vi "Day 10-2.vi"() -> ()   [LabVIEW 2019, in "Day 10.lvlib"]
uses:
  Day 10.lvlib
panel:
  out "Result":u64
  in  "String":string="[[{(<({[(([[([()<>][()<>])]][<{[[]<>]}<<[]{}>>>])[({<[{}[]]<{}<>>><{()[]}[{}[]]>}<<(<>[])[[]{}]>{(<\n{{{[[<{<{({({(<>{})}<(()[])([]<>)>)})(<[([{}()]([]{}))[([][])([]<>)]]((<{}<>>[[]{}])({<>()}{()}))>\n[(<<[(<[[[<{(([]{})){<{}{}>{()<>}})><(<[()()][<>]>([[]]))[(([]<>)(<><>))((<>)({}[]))]>]{<<{{()[]}<[]<>>}\n{{({{{([<((<[[<>[]](<>[])]><<(()<>)<<><>>>{(()<>)(<>{})}>))>]({(([{{()()}>{{{}{}}{<><>}}]{({()<>\n<<{(<<{<<{([{{(){}}{()()}}{<[]{}>(<>{}))][({<>{}}[[]<>])<{{}{}}{{}()}>])[<<{{}{}}[()[]]>{{\n[[<{[<((<[[{{{{}{}}{{}[]}}}[[<{}<>>]]]({<([][]){{}<>}>((()<>)<<>[]>)})]><[({{<{}()>{()()}}})]{(<({[]{}}[{\n<<[{([[[[[<{[([]())({}[])]{[{}[]]}}<(<[]{}>({}{})){{[]<>}[()]}>>{(<{[]}[<>[]]>)}][(([[{}[]]<[]\n[(<[<{{((<{<[<{}[]>[<>{}]][<{}<>>]><<({}[])[[]<>]>}}>)<(([{<{}<>>(()[])}[[{}()]([])]]<<{<>()}({}{})>\n<{{[[<(<<<([({{}())([]{})){<()<>>{<>{}}}]<{[[]{}][[]<>]}{<{}()>{[]()}}>)<<{(<>())[<><>]}[{{}[]}(<>(\n{{{{<{{<{<<[[[{}()]<[][])]<{(){}}{[]{}}>][{<[]()>{<>{}}}]>><{(<<<>[]>{(){}}>{{[]()}[<><>]}){(<{}()>){[[][]](\n{(<{{([[(<{[((()<>){()()})<[<>{}]{()}>]<{[()[]]}>}([{<()>{{}[]}}[([][]){()[]}]]{{<<>[]>}{([]{}){<><>}}})\n[(((({[{<<{[{([]())(<>[])}[<{}()>{()()}]]}>>[<[[{{{}()}{()<>}}(<()<>>[{}[]])]{[({}<>)<<>>]}]<({<<><>\n<([[[((<[<<((<[][]>))<<{[][]}>>>{<([()()>)>}><([[[()[]]({}())]({<>{}}{()[]})]{{{<><>}[[]()]}[[[]\n(((<({([[({{({[][]})(({}())[()<>])}(<[[][]]>(<{}>[<>{}]))})](<{((<<><>>[()()]){<[]<>>[[]<>]})}([<\n[[{[[{[[{[{{[<{}()><()[]>]}}]<<{{<<><>>{{}{}}}[(<>{})(()())]}[{([]<>)[{}()]}<[[]][()()]>]><<{{[]{}}\n((<<((<(<[{[({()<>}{()()}){<{}{}>}]}[{<[<>()][[]()]>}]]{[{[<()>{[]{}}]}<{[{}{}}}[([]{})(<><>)]>](({(<>{})\n[[<[<({[[<<{[[()()]{(){}}]<[{}<>](()())>>(<[()[]][[]()]>)>[{(([][])([]{}))}[<<<><>><()<>>>(<<>[]>)]\n[({(<{(<{[{[{([]){{}{}}}(<[][]>(<>[]))](<{<>[]}<[]()>>{<()><{}>})}{[([<>{}]{[]()})[(<>{})<[]()>]][{[()<>\n[[<<{[(<({(((([]{})[[][]])<<{}{}>{[]()}>))})<[(<<(<>[])<[]()>><((){})[()<>]>>{<({}[])>{<<>{}>{(){}}}}\n<<([[({(<{<[[({}()){()[]}]]>((<<()[]>(<>{})>(([]())))(((()<>)({}[]))))}>{<{((([])<()[]>)<({}())<()<\n<<({[<{<({{{{[()()]<<>[]>}[{{}<>}[()()]]}{(([]()))})})[[[{[<<>[]>[<>()]]<{[]{}}[<>{}]>}]([{{[][]}{\n{((((([[([<{([<>{}]<{}[]>){({}())[{}[]]}}{(<()()>({}[]))<{<><>}(<>[])>}>([<{()<>}[()[]]><[()<>]>]{[{\n{[((((({<[{<{[(){}][[]()]}[({}[])]>{[[<>{}]{{}}]{[<>[]]<<>[]>}}}({[([]{})]{[[]<>]<[]{}>}}(<(()[])[{}()]\n((<<{<{{{<(<<[<>()]{{}<>}>({<>{}}[[]()])>(<<{}<>>({}<>)><[{}<>]{(){}}>))<(((()[])([]())){(<\n{(<(<([{{{((([<>[]]([]<>))({<>[]}<<>[]>)}{<(<><>)<<>{}>>(({}[])(()<>))}){[{{{}{}}}]{[<{}()>(<>{})][{[]}]}\n{{{([([(<[<[{<()>{()()}}<[()()]<<><>>>]{<<()<>>>(((){}){()<>})}>{<{({}[])<<><>>}((()())<{}{}>)>\n{(({(<<([[({<{[][]}<<><>>>}(<({}<>){{}<>}>{<<><>>(<>())}))<{{[{}<>]<[]()>}<<{}{}>>}[{<{}[]><(){}>}{\n[[[([[(([<[<{<<>{}><{}[]>}>((<[][]>[{}[]]))]{({<<><>>[()[])}[{{}()}<{}>])}>]){[{{((<<>{}>([]<>))([\n([<<<[(<(<{[[({}{}](<>)]{{{}<>}({}{})}][({()}{[]()})[({})]]}{<[(<><>)({}{})]<{<>}{[]}>>}>)>){{<[(<{(()()\n{{{<{(<(([<<<{{}[]}[<>{}]}>([<<>()>{<>()}]<<<><>>[{}<>]>)>{[([<>()]{()[]}){{<>{}}[<>[]]}]}][(<[(()\n<<<[[{(([<<{{(()())[{}[]]}{[[]<>]<<>>}}[(<<>><{}<>>){{{}[]}[{}()])]>([(<{}()>[[]()])[(()())\n{{{([[[<{(<<{[[]()](<>{})})[(<[]{}><[]{}>)[<[]{}>{{}()}]]>[[[(()()){{}{}}][[<>[]](())]]<([{}()][{\n([{{([[[({[(((<>)(()<>)){[{}{}](()())}){(((){})([]()))[(<>{})<[][]>]}]([({[]()}[(){}])<[{}()>(()<>)>\n[[[<<(({<<(([({}[])<(){}>][[{}]([]())])<{{[]()}[[]]><{<><>}<()[]>>>)>{<{<[[][]]<{}<>>>([[]<>]{{}<\n[[[<[<([{<[{{{()<>}({}<>)}}(<{{}<>}{[]()}>[<()())(<>())])]>[[(<{()}<[]()>><[()[]]<<>{}>>){<[()<\n{{(<({((<[<<[([][])<[]<>>](<<>[]>)>>{<([(){}]{[]{}})>{[({}<>)]<[(){}]{{}}}}}]>)[[[[<{<[][]>(\n[[[[{{{{([(((({}<>){()()})[{()()}([]<>)])[{<{}{}><[]{}>}([()<>][[]()])])]))}(<[[[{[[()[]]<()[]>]}]{((\n({{[(((([<({{(<>())<{}()>}([{}{}]<{}{}>)}[{[{}{}]}<[[]]<()[]>>])[([<{}{}><[]{}>])<<[(){}]({}{}\n(<<({<({[({[{{()[]}[()<>]}<{<>{}}({}{})>](<{<>{}}>[{{}<>}{(){}}])})(({<<{}[]>{<>()}>}{{<<>()>\n[[[[<<<({<({({[]}[[]{}])(<{}()>[{}{}])}[[({}())][{<>{}}{[]<>}]])>})<([<(<(()[])([]())>)<[[{}[]][{}<>]][[(\n{<{<{<[[{[[<(([]{})){[()[]][{}[]]}><[{<>{}}({}{})]{({}())<<>[]>}>]]}(([<[{<>()}{(){}}]<<[]{}>(()())>>]\n{<<<{<{<(<{([(<>)<[][]>][(()[]){{}<>}])}(((({}<>)<[][]>){([]<>){()<>}})<<<<>()>{{}()}>{<[]()><[]()>}>)})[<{\n([<<[[{{<[{(<{[]()}>)<<<<>()>([]<>)>>}]{(({{<>()](()<>)}(({}())[[]()])))}>{(<[<(<><>)[{}<>]\n[{<<{[[<[<<{{<<>()>}[[{}[]]({}{})]}([[<>[]]][(<><>)<()()>])>[({[<><>][[]<>]})({<[][]>(()<>)})]>}>][{(([<[{\n{([[[<[(([[<<<()<>>[<>()]>[<()<>><(){}>]>[<<[][]>(<><>)>]][(([<>()]<<>()>))<([{}()]{{}{}}){<()[]){[]()}}>]]{[\n{{<<[<{{([({[([]<>)[{}()]]{[()[]>[()()]}}<[[<>{}](<><>)]>)[<(<<><>><[]{}>)([<>{}])><<{[]}[{}()]>{<<>{}>[<>[]\n{{<(<<((<[<<<[{}[]]<<><>>>[({}[]){{}()}]>>]>){(<([(<<>[]><{}>)({<><>}<{}[]>)]{{([]{}>(()())}\n[(<<<{[<([[(({()()}<{}[]>){[{}<>]([]<>)})({(<>[])(()<>)}[([][])<())])]])({[<(([][]){()()})>{[[(\n[<[[(({[<<([{({}[])[{}{}]}{<<>[]>[{}{}]}])[[({{}}<[]>){<[]()>{{}{}}}]<{[<>[]](<>())}<[()()][()<>]>>]>(<[[[[\n{<{[([[<<<{<<({}{})(<>())>{<<><>><{}{}>}>{({()()}<{}()>)<(<>{}){<>[]}}}}({[{[]{}}{()<>}](<<><>>(\n{{<<([{([[(([{()<>}<(){}>]<<()()>(()<>)>)({[{}()]}<<()[]><()()>>))][[<(((){})<[][]>)><(<<><>>\n{(([{({<{[({[(<><>)(()()]]<[<>[]][{}<>]>})]}>{(([[(<()[]>(()<>)){{[]<>}(<>())}]([<[]()>[{}[\n{{({{{<{{{[([[<><>]]<{[][]}[[]<>]>)(<<<><>><<><>>>[(()())({}<>)])]((<(<><>)<(){}>>[{{}{}}[{}<>]])([<()[]>\n{(<<{{<<{{{{<<[]<>>[{}()]><<()[]>{{}[]}>}}}}([({<<{}{}>[()]>[[{}[]]<[]{}>]}(<{()()}<()[]>>))]{\n{<<([((<<[<{({{}[]}<()()>)(([]{})<{}[]>)}<(((){})[()<>])>><(<(<><>)<<><>>>){[((){})([]<>)](([][])[<\n<{[{<{<<({<<([{}()]{[]{}})[({}())<{}()>]>>[[[(()[])[()<>]](<[][]><{}()>)][(([]()]([]))]]})>>{<[<[((<{}<>>{(\n[{[[[({<<[[([{<>{}}[[]]]<<{}<>><[]<>>>)(<<{}()>[()<>]>[<(){}>])][<{<()()><<>[]>}<[[][]][<>()]>><[[{}()](<>)\n<{{[{[{[([[[([<><>]({}[]))([[][]](<>{})}][[{[]()}{{}()}][{[][]}<{}<>>]]][(({[]<>}[<>()])[<()<>><[][]>])<(({}\n{(({[{(<[<(<[{<><>}<{}[]>]<[{}<>]((){})>>([{()}(<><>)])){<[<()<>>[{}()]]({<>{}}(<><>))>{{(<\n<<[[(<{<({<<[[<>()]((){})]>{[({})<{}<>>]((<>{}){[]<>})>>})>}>({{(<<{([()[]])[{{}[]}(<>[])]}>>)}<((<<<\n[[([{{((<(<({{[]<>}}<{<>()}([]())>)<[<<>()>(<>{})][[()()]<<>{}>]>>)>(<[[{[{}{}]({}[])}({{}{}}[[]()\n<{[[{[([<([{<<()()>><<<>[]>>}][[((<>)(<><>))<({}{})<()<>>>]<{[<>()]<[]{}>}>])({[[{[]{}}]]}{({[<>()\n<<[<{<([([<({<(){}>{[]()}}<<{}<>><[]<>>>)>{{<[(){}]{<>()}>(<<>()>[{}<>])]}](<(<(()())<<><>>\n[{[<[<[<<(<[(<<>{}>)[<{}{}>({}{})]]})>[[(((<<>[]>[<>()])<{(){}}<(){}>>){{(<><>)}[(<>()){{}<>}]})\n{<{<({{(<(<([[<>()][[]()]][(()[])[[]<>]])[([[]{}]{{}<>})]>[[<({}()){<><>}><{()[]}({}())>]([{<>{}}\n({(([(<[[{{<([[]()]{{}{}})[{{}{}}[{}<>]]>[{([]<>)(()())}(<<><>>{<>{}})]}<<({()()}{()<>})[(<>\n[<[<((({{<{([({}())([]{})]<(()())(<>())>)({<()[]>{<>[]}})}<[([()<>]{{}<>})](<{[]()}(<>())>)>>[({[([])(\n({[<[(<((<{(<[()[]>[{}<>]>)<{<[]<>>{<>[]}}(({}{}))>}{{<[[]{}][{}{}]>{(())<[]()>}}}><<<{(<>[])<[]()>}({[][\n(<<<({({<[[<<(<><>}<()<>>>{<{}<>><[]<>>}>[<<[]<>>(()[])>{<()()>}]]]{{(([<>[]]<[]{}>){({}{})([][]\n({<[[<[({[{<{(()<>)}[(()[])<<>{}>]>}({{(<><>)[<><>]}[{[]()}<(){}>]}{{[()()]<(){}>}[[{}[]]([]{})]})]([[<{{}()}\n[[[(<({(({{{<{()<>}[<>{}]><<[][]>({}[])>}[[[{}{}]<<>{}>][[(){}]]]}[<([{}{}][[]])[{<><>}[()[]]]>]}<<[({{\n[<[[{[(([[<{(<{}{}>)}(<{(){}}([][])>{<(){}><<>{}>})>([([{}{}])(<[]><(){}>)])][({<<{}<>><[]<>>>[[[]{}]{[]{}}]\n[{{[(<<{{{[([(()())<<><>>])<([()()]((){}))<([][]){[]<>}>>]{<<{(){}}(<><>)>({()<>}<()[]})>}}}}[{{<<\n<[{[(({({<(<<<{}{}>{{}{}}>{([])({})}>{[{<>>(<>)]{[<>{}]<{}<>>}})[<({{}[]}<{}{}>)<([]())({}())>>({<[]\n(<[<({[{{(((({{}[]}{{}<>}){(<>[])})[[({}<>)[[]<>]]<[{}]{[][]}>])(<[(<>()){<>()}]<(<><>){(){}}>>\n[([{([{[<{<[<(<>{}){{}[]}>{([][]){()}}]{[<[]{}><<>{}>]{[(){}){[]{}}}}>([<[{}]<{}[]>>{<[][]>{()[]}}][{{<>()}{{\n<{{(({({[<(({({}[]){{}<>}}[(<>()){[]{}}]))[[<{()()}[{}{}]>(<{}{}>(<>[]))]<<{()()}<{}{}>><{<><>}<<>[]\n{{[[<[<[{[<{{[[]<>]<[]>}[({}{})(<>)]}>](<<((<>)<[]<>>)[<{}()><<>[]>]>[<{<>()}<(){}>>[[()<>]]]>(<[{\n({[<(<{<[<<<(<<>()><[]<>>)<<()<>>({}[])>>(<[()()]{<><>}>)>>]>(<<({[<{}[]>{()}]}<<{()<>}({}())>({[]<>}([]()))>\n<{<{{[({{(<{<<<><>><(){}>>[([][])([]{})]}<{([][]){{}}}<<[]()>([][])>>>[<{{[]()}[()<>]}<[<>{}]([]{})>>])\n{({[{(<[<<<<(([]<>)<{}{}>)>((({}{})<{}<>>)<<{}{}>>}>{{[<()()>[{}()]]}((<<>()>[(){}])<{[]<>}[<>{}]>)}>>{<<{\n((([<[[[<{{<<<{}[]><<>{}>>(([]<>)[[]])>((<{}[]><{}>)(({}[])[()[]]))}{{<(<>[])(<><>)>(<<>[]\n[[([{<(<(<[({[[][]]{()<>}}{{<>[]}<[][]>})]>)<{[((((){})([]<>))[<<><>>(<><>)]>[{<{}[]><[][]>\n[<<(<(({{{<((([]())[<>{}])<[[][]]{()()}>)><[<((){})<()()]>[<[]>[(){}]]]({([]())([]{})}([<>(\n(<{<<{<((({(<{(){}}[()<>]>{[[]<>][()[]]})<<{[][]}{{}[]}>[(<><>)<{}{}>]>}(<[{{}<>}{[]()}]({()[]}((\n<[[([<<[{{<(<[()[]]{<><>}>([<>[]]<{}[]>))[({{}()}<[]<>>)<(<>{})>]>{{{<<>{}>(<>)}<{<>()}[<>()]>}<[<<>()\n[[((<({<[{{<[[[]()][<>]](<()()>[{}<>])>{<(()<>)>([()<>]{()[]})}}{[[(()<>><[]<>>]]<{(<><>){{}<>}}\n[<{([{[{<<<(<[<><>]({}())>{([]<>][[]{}]})[<{[]<>}[<>{}]>[<[][]>]]>>({([(<><>){<>{}}][{{}[]}({}<>)\n{({{<[([{([<<{<>()}>[{<>[]}[{}[]]]>](<{{[]{}}[{}<>]}({<>[]}[{}[]])>[<([][])({}{})><<{}()>(()<>)\n(<({[<(<[<[{([[]{}][{}[]])([{}[]])}{({<>[]}{()[]})[[<><>](()<>)]}]><(({[()[]]}([{}()][{}{}]))<[(()<>)]>)[[<\n<(<(<<({({[<{<<><>>[()<>]}{<[]()><<><>>}>[(([][])<{}[]>)(({}{})<<>()>)]](<<(<><>){[]<>}>([[][]][<>()])>{<(\n[({<[[<{[[{[{{<>()}{{}[]}}](([{}[]}{[][]})<{<>[]}({}<>)>)}{[(([]{})<{}[]>)<<{}>{(){}}>]}]<[\n<[({<<[[({{{((<><>)<[]<>>)<<{}><{}<>>>}(([(){}]{()})[{[][]}[[]<>]])}}[[<[<()[]>[{}()]]><{<{}<>><<>[]>}{[[]\n<[{[[[[[<{[<([<>()]([]{}))<{[]{}}<[][]>>>([{[]<>}([]<>)]{[{}()][<>{}]}}]<[[(<><>)[{}{}]][(()(\n{<{{[<({{<[([{()()}[{}<>]]{({}())<(){}>})[[{(){}}<[]<>>}<(<>()){{}{}}>]]{{(([]{})[[]()])[{{}{}}[[]{}]]}{<[\n(([<([<<{[{{[({}{})][(<>{})]}}]{{([<<>{}>(<>())])}}}>[{<<(({{}<>}<<>[]>){({}())<{}()>})><(<[()<>]><{()<>}<\n[<[{[[[({[{[(((){}){(){}}){{<><>}{{}[]}}]<{({}()){<>{}}}>}<{[{[]{}}({}{})])>]}{(<(((()[]){{}[]})[<()<>\n({<<([{{{{({[{<>[]}[{}{}]]{<[]{}><{}{}>}}[<[<>()](<><>)><[{}{}]>])(<{[<>()]<<>()>}<(<>[])>>(([()"
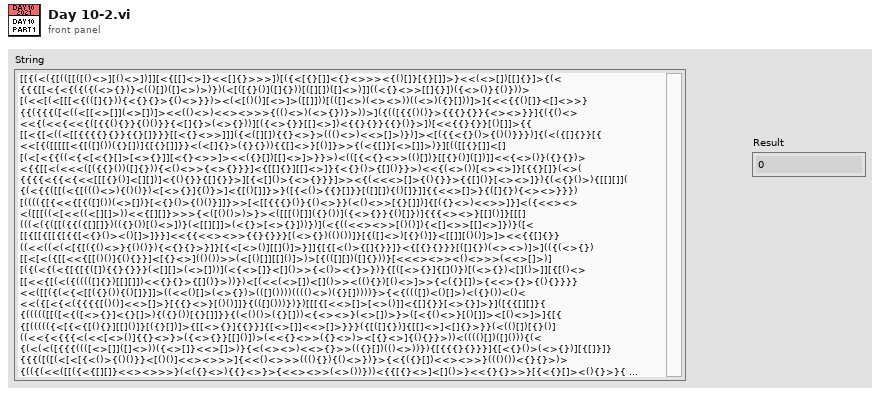
[diagram p1: front panel]
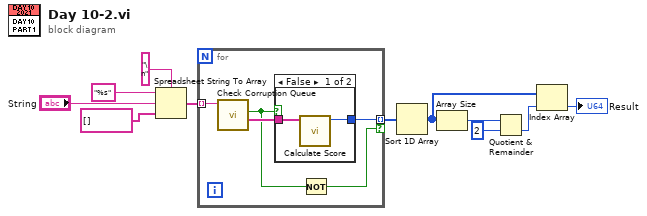
[diagram p0: block diagram]
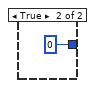
[diagram p2: hidden frame]
diagram:
  n1 = Spreadsheet String To Array(delimiter (Tab)="\n", format string="%s", spreadsheet string="String", array type (2D Dbl)=string[] []) -> (array=w7:string[])
  n2 = for {
    tunnel: w7 -> [w16] mode=indexing
    tunnel: [w14] -> w1 mode=indexing if=w12
    n3 = call "Check Corruption Queue.vi"("input string"=w16) -> ("Remaining string"=w15:string[], "Corrupted?"=w13:bool)  [unwired: 7 in, 2 out]
    n4 = case shown="False" w13 {
      tunnel: w15 -> [w18 _]
      tunnel: [w17 u64 0] -> w14
      frame False {
        n5 = call "Calculate Score.vi"("Remaining string"=w18) -> ("Score"=w17:u64)  [unwired: 10 in]
      }
      frame True {
      }
    }
    n6 = Not(x=w13) -> (.not. x?=w12:bool)
  }
  n7 = Sort 1D Array(array=w1) -> (sorted array=w4:u64[])
  n8 = Array Size(array=w4) -> (size(s)=w6:i32)
  n9 = Quotient & Remainder(x=w6, y=2) -> (floor(x/y)=w3:i32)  [unwired: 1 out]
  n10 = Index Array(array=w4, index=w3) -> (element=→"Result":u64)
